vi "Backup Local Files.vi"(6 "Error Message in":string, 8 "Error In":errorcluster, 10 "Local Version Array":i32[](array[numeric]), 11 "Server Files Cluster":T1) -> (0 "Error Out":errorcluster, 4 "Error Message out":string)   [LabVIEW 2019]
uses:
  <userlib>/_OpenG.lib/lvzip/lvzip.llb/ZLIB Open ZIP Mode__ogtk.ctl
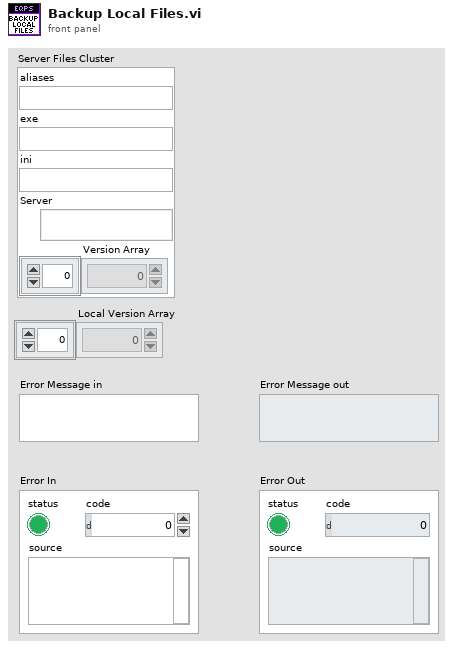
[diagram p1: front panel]
types:
  T1 = cluster{"aliases":string, "exe":string, "ini":string, "Server":path, "Version Array":i32[]}
  T2 = typedef "ZLIB Open ZIP Mode__ogtk.ctl" = enum16{"create new", "append to end", "append to archive"}
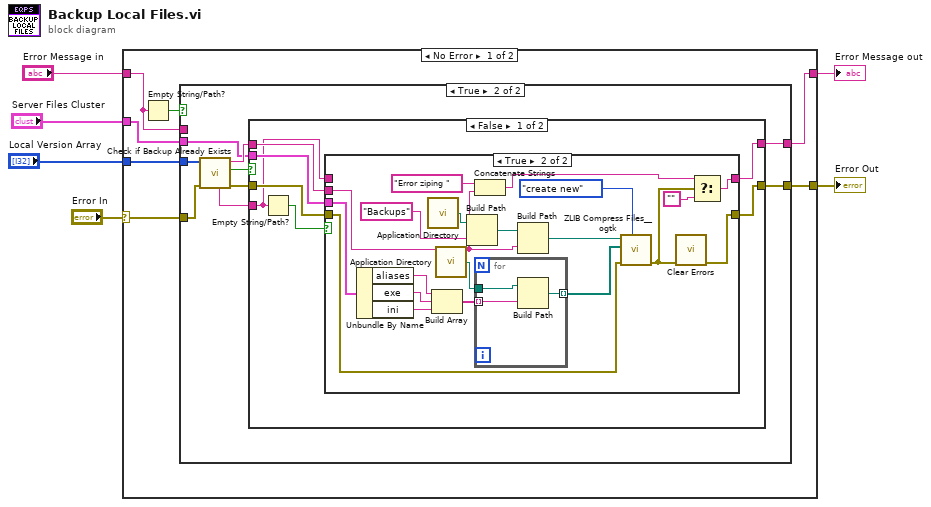
[diagram p0: block diagram]
diagram:
  n1 = case shown="No Error" "Error In" {
    selector: "Error In" -> [w9 w60]
    tunnel: [w10 w60] -> w5
    tunnel: [w12 w59] -> w4
    tunnel: "Error Message in" -> [w11 w59]
    tunnel: "Local Version Array" -> [w8 _]
    tunnel: "Server Files Cluster" -> [w7 _]
    frame No Error {
      n2 = Empty String/Path?(string/path=w11) -> (empty?=w13:bool)
      n3 = case shown="True" w13 {
        tunnel: [w15 w17] -> w12
        tunnel: w11 -> [w15 _]
        tunnel: [w14 w18] -> w10
        tunnel: w9 -> [w14 w24]
        tunnel: w8 -> [_ w23]
        tunnel: w7 -> [_ w16]
        frame False {
        }
        frame True {
          n4 = call "Check if Backup Already Exists.vi"("Error In"=w24, "Local Version Array"=w23) -> ("Error Out"=w22:errorcluster, "File Exists"=w21:bool, "Filename"=w20:string, "Error Message out"=w19:string)  [unwired: 6 in]
          n5 = case shown="False" w21 {
            tunnel: w22 -> [w30 w58]
            tunnel: w20 -> [w28 _]
            tunnel: w19 -> [w25 w57]
            tunnel: [w29 w58] -> w18
            tunnel: [w26 w57] -> w17
            tunnel: w16 -> [w31 _]
            frame False {
              n6 = Empty String/Path?(string/path=w25) -> (empty?=w27:bool)
              n7 = case shown="True" w27 {
                tunnel: w31 -> [_ w53]
                tunnel: w30 -> [w32 w42]
                tunnel: [w32 w37] -> w29
                tunnel: w28 -> [_ w39]
                tunnel: [w33 w35] -> w26
                tunnel: w25 -> [w33 _]
                frame False {
                }
                frame True {
                  n8 = Unbundle By Name(w53) -> ("aliases"=w51:string, "exe"=w52:string, "ini"=w50:string)
                  n9 = call <vilib>:"Application Directory.vi"() -> ("Application Directory"=w47:path)
                  n10 = Build Array(w51, w52, w50) -> (w49:string[])
                  n11 = call <vilib>:"Application Directory.vi"() -> ("Application Directory"=w48:path)
                  n12 = Build Path(base path=w47, name or relative path="Backups") -> (appended path=w45:path)
                  n13 = Concatenate Strings("Error ziping ", w39) -> (w38:string)
                  n14 = for {
                    tunnel: w49 -> [w56] mode=indexing
                    tunnel: w48 -> [w55]
                    tunnel: [w54] -> w43 mode=indexing
                    n15 = Build Path(base path=w55, name or relative path=w56) -> (appended path=w54:path)
                  }
                  n16 = Build Path(base path=w45, name or relative path=w39) -> (appended path=w44:path)
                  n17 = call <userlib>:"ZLIB Compress Files__ogtk.vi"("append (create new)"=ZLIB_Open_ZIP_Mode__ogtk."create new", "error in (no error)"=w42, "file names"=w43, "archive name (file dialog)"=w44) -> ("error out"=w36:errorcluster)  [unwired: 6 in, 1 out]
                  n18 = call <vilib>:"Clear Errors.vi"("error in (no error)"=w36) -> ("error out"=w37:errorcluster)  [unwired: 5 in, 1 out]
                  n19 = Select(t=w38, s=w36, f="") -> (s? t:f=w35:string)
                }
              }
            }
            frame True {
            }
          }
        }
      }
    }
    frame Error {
    }
  }
  "Error Out" <- w5
  "Error Message out" <- w4
